vi "SaveLotData.vi"(8 "error in (no error)":errorcluster, 11 "EpiWrapper in":refnum<class "EpiWrapper.lvclass">) -> (0 "error out":errorcluster, 3 "EpiWrapper out":refnum<class "EpiWrapper.lvclass">)   [LabVIEW 2012, in "EpiWrapper.lvclass"]
uses:
  EpiWrapper.lvclass
  EpiWrapper.lvclass/EpiWrapper.ctl
  LotData.lvclass
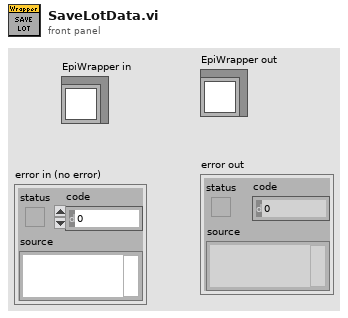
[diagram p1: front panel]
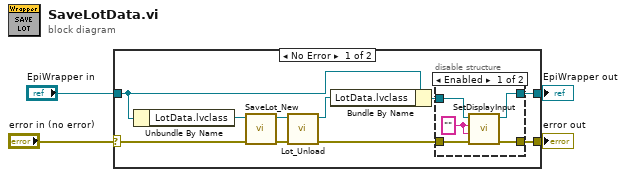
[diagram p0: block diagram]
diagram:
  n1 = case shown="No Error" "error in (no error)" {
    selector: "error in (no error)" -> [w12 w23]
    tunnel: [w5 w23] -> w3
    tunnel: [w6 w22] -> w1
    tunnel: "EpiWrapper in" -> [w13 w22]
    frame No Error {
      n2 = Unbundle By Name(w13) -> ("LotData.lvclass"=w14:refnum<class "LotData.lvclass">)
      n3 = call-dynamic "SaveLot_New.vi"("error in (no error)"=w12, "LotData in"=w14) -> ("error out"=w10:errorcluster, "LotData out"=w11:refnum<class "LotData.lvclass">)  [unwired: 7 in, 1 out]
      n4 = call-dynamic "Lot_Unload.vi"("error in (no error)"=w10, "LotData in"=w11) -> ("error out"=w8:errorcluster, "LotData out"=w9:refnum<class "LotData.lvclass">)  [unwired: 8 in]
      n5 = Bundle By Name(cluster=w13, "LotData.lvclass"=w9) -> (w7:refnum<class "EpiWrapper.lvclass">)
      n6 = disable-structure shown="Enabled" {
        disable-tunnel: w8 -> [w18 w20]
        disable-tunnel: w7 -> [w17 w21]
        disable-tunnel: [w16 w21] -> w6
        disable-tunnel: [w15 w20] -> w5
        frame Enabled {
          w19 = "" ("Wafer ID")
          n7 = call-dynamic "SetDisplayInput.vi"("error in (no error)"=w18, "Test"=w19, "Wafer ID"=w19, "EpiWrapper in"=w17) -> ("error out"=w15:errorcluster, "EpiWrapper out"=w16:refnum<class "EpiWrapper.lvclass">)  [unwired: 6 in]
        }
        frame Disabled {
        }
      }
    }
    frame Error {
    }
  }
  "error out" <- w3
  "EpiWrapper out" <- w1
